vi "TCP 읽기.vi"() -> ()   [LabVIEW 2014]
panel:
  out "웨이브폼 그래프":dbl[](graph)
  out "에러 출력":errorcluster
  in  "정지":bool
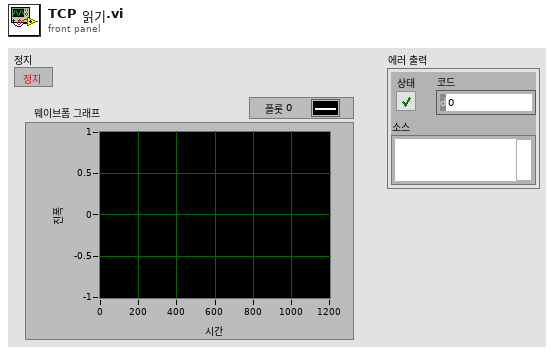
[diagram p1: front panel]
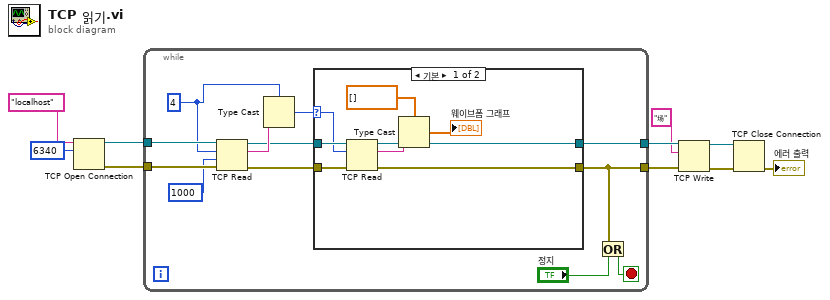
[diagram p0: block diagram]
diagram:
  n1 = TCP Open Connection(address="localhost" ("주소"), remote port or service name=u16 6340 ("원격 포트 또는 서비스 이름")) -> (connection ID=w8:refnum<k5>, error out=w7:errorcluster)  [unwired: 3 in]
  n2 = while {
    tunnel: w8 -> [w22]
    tunnel: w7 -> [w21]
    tunnel: [w14] -> w5
    tunnel: [w12] -> w6
    stop <- w13 stop-if-true
    w16 = 4 ("읽을 바이트")
    n3 = TCP Read(connection ID=w22, bytes to read=w16, error in (no error)=w21, 9:1000 ("타임아웃 ms (25000)")) -> (connection ID out=w15:refnum<k5>, data out=w17:string, error out=w19:errorcluster)  [unwired: 1 in]
    n4 = Type Cast(type=w16, x=w17) -> (*(type *) &x=w18:i32)
    n5 = case shown="기본" w18 {
      selector: w18 -> [w28 _]
      tunnel: w19 -> [w29 w31]
      tunnel: w15 -> [w30 w32]
      tunnel: [w27 w32] -> w14
      tunnel: [w26 w31] -> w12
      frame Default {
        n6 = TCP Read(connection ID=w30, bytes to read=w28, error in (no error)=w29) -> (connection ID out=w27:refnum<k5>, data out=w25:string, error out=w26:errorcluster)  [unwired: 2 in]
        n7 = Type Cast(type=dbl[] [], x=w25) -> (*(type *) &x=→"웨이브폼 그래프":dbl[])
      }
      frame ..0 {
      }
    }
    n8 = Or(x=w12, y="정지") -> (x .or. y?=w13:bool)
  }
  n9 = TCP Write(connection ID=w5, data in="场" ("데이터 입력"), error in (no error)=w6) -> (connection ID out=w2:refnum<k5>, error out=w3:errorcluster)  [unwired: 1 in, 1 out]
  n10 = TCP Close Connection(connection ID=w2, error in (no error)=w3) -> (error out=→"에러 출력":errorcluster)  [unwired: 1 in, 1 out]
